vi "DelayPeriod.vi"(8 "error in (no error)":errorcluster, 11 "TrialBasedExperiment in":refnum<class "ClassDiscrimination.lvclass">) -> (0 "error out":errorcluster, 2 "Timeout":dbl, 3 "TrialBasedExperiment out":refnum<class "ClassDiscrimination.lvclass">)   [LabVIEW 2014, in "ClassDiscrimination.lvclass"]
uses:
  ClassDiscrimination.lvclass
  ClassDiscrimination.lvclass/ClassDiscrimination.ctl
  Trial Based Experiment Statechart/MatlabExperiment/MatlabExperiment.lvclass
  Matlab API/Matlab API.lvlib
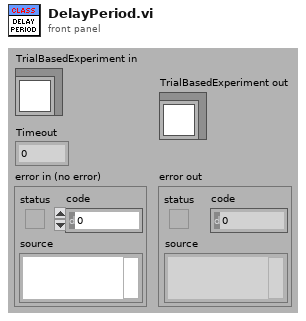
[diagram p1: front panel]
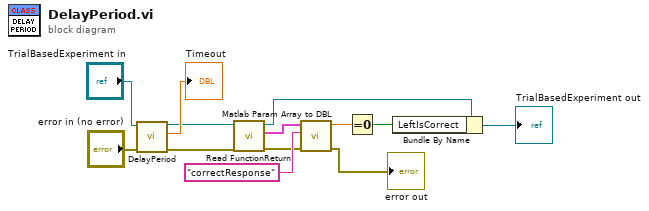
[diagram p0: block diagram]
diagram:
  n1 = call-parent "DelayPeriod.vi"("error in (no error)"="error in (no error)", "TrialBasedExperiment in"="TrialBasedExperiment in") -> ("error out"=w9:errorcluster, "Timeout"=→"Timeout":dbl, "TrialBasedExperiment out"=w10:refnum<class "ClassDiscrimination.lvclass">)  [unwired: 7 in]
  n2 = call-dynamic "Read FunctionReturn.vi"("error in (no error)"=w9, "MatlabExperiment in"=w10) -> ("error out"=w6:errorcluster, "FunctionReturn"=w7:cluster{"Name":string, "Data":variant}[], "MatlabExperiment out"=w4:refnum<class "ClassDiscrimination.lvclass">)  [unwired: 7 in]
  n3 = call "Matlab Param Array to DBL.vi"("error in (no error)"=w6, "Name"="correctResponse", "Matlab Param Array"=w7) -> ("error out"=→"error out":errorcluster, "data"=w3:dbl)  [unwired: 7 in]
  n4 = Equal To 0?(x=w3) -> (x = 0?=w2:bool)
  n5 = Bundle By Name(cluster=w4, "LeftIsCorrect"=w2) -> (→"TrialBasedExperiment out":refnum<class "ClassDiscrimination.lvclass">)
